vi "BuildTriggerArray for Closed IPG.vi"(0 "CBC Trigger Level":dbl, 1 "Load Resistance (Ohms)":dbl, 2 "Target Stim Current (Amps)":dbl, 3 "Krec Value":i32, 4 "Recovery Mode (T=Active)":bool) -> (5 "Pulse Triggers":T1(array[cluster]))   [LabVIEW 2010]
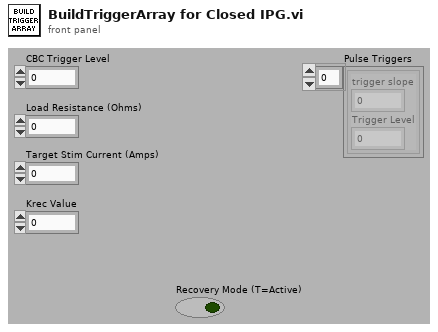
[diagram p1: front panel]
types:
  T1 = cluster{"trigger slope":u16, "Trigger Level":dbl}[]
  T2 = cluster{"trigger slope":u16, "Trigger Level":dbl}
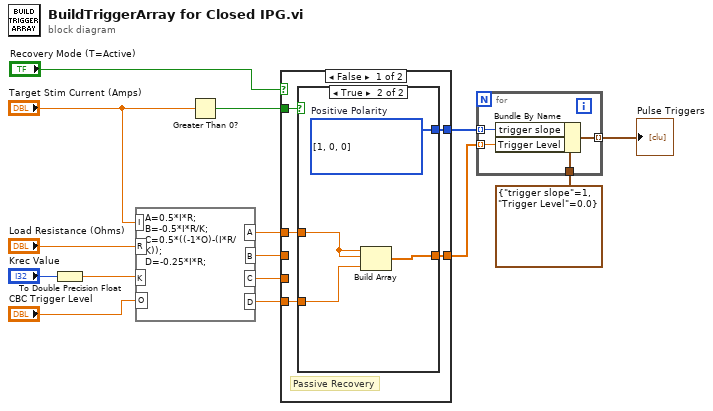
[diagram p0: block diagram]
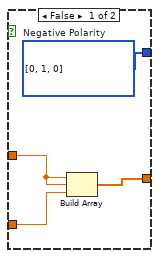
[diagram p2: hidden frame]
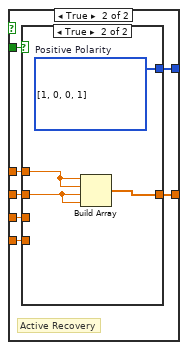
[diagram p3: hidden frame]
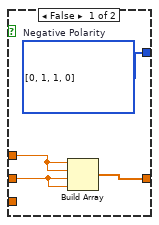
[diagram p4: hidden frame]
diagram:
  n1 = To Double Precision Float(number="Krec Value") -> (double precision float=w8:dbl)
  n2 = formula code="A=0.5*I*R;\nB=-0.5*I*R/K;\nC=0.5*((-1*O)-(I*R/K));\nD=-0.25*I*R;"("R"="Load Resistance (Ohms)", "I"="Target Stim Current (Amps)", "K"=w8, "O"="CBC Trigger Level") -> ("A"=w5:dbl, "B"=w4:dbl, "C"=w3:dbl, "D"=w2:dbl)
  n3 = Greater Than 0?(x="Target Stim Current (Amps)") -> (x > 0?=w14:bool)
  n4 = case shown="False" "Recovery Mode (T=Active)" {
    tunnel: [w19 w35] -> w11
    tunnel: w14 -> [w20 w34]
    tunnel: w5 -> [w18 w33]
    tunnel: w4 -> [_ w32]
    tunnel: w3 -> [_ w31]
    tunnel: w2 -> [w17 w30]
    tunnel: [w16 w29] -> w1
    frame False {
      # "Passive Recovery"
      n5 = case shown="True" w20 {
        tunnel: [w24 w28] -> w19
        tunnel: w18 -> [w23 w27]
        tunnel: w17 -> [w22 w26]
        tunnel: [w21 w25] -> w16
        frame False {
          w24 = u16[] [0, 1, 0] items=["Falling Edge", "Rising Edge"]  # Negative Polarity
          n6 = Build Array(w23, w23, w22) -> (w21:dbl[])
        }
        frame True {
          w28 = u16[] [1, 0, 0] items=["Falling Edge", "Rising Edge"]  # Positive Polarity
          n7 = Build Array(w27, w27, w26) -> (w25:dbl[])
        }
      }
    }
    frame True {
      # "Active Recovery"
      n8 = case shown="True" w34 {
        tunnel: [w39 w43] -> w35
        tunnel: w33 -> [w38 w42]
        tunnel: w32 -> [w36 w40]
        tunnel: w31 -> [_ _]
        tunnel: w30 -> [_ _]
        tunnel: [w37 w41] -> w29
        frame False {
          w39 = u16[] [0, 1, 1, 0] items=["Falling Edge", "Rising Edge"]  # Negative Polarity
          n9 = Build Array(w38, w38, w36, w36) -> (w37:dbl[])
        }
        frame True {
          w43 = u16[] [1, 0, 0, 1] items=["Falling Edge", "Rising Edge"]  # Positive Polarity
          n10 = Build Array(w42, w42, w40, w40) -> (w41:dbl[])
        }
      }
    }
  }
  n11 = for {
    tunnel: T2 {"trigger slope"=1, "Trigger Level"=0.0} -> [w47]
    tunnel: w11 -> [w46] mode=indexing
    tunnel: w1 -> [w45] mode=indexing
    tunnel: [w44] -> w13 mode=indexing
    n12 = Bundle By Name(cluster=w47, "trigger slope"=w46, "Trigger Level"=w45) -> (w44:T2)
  }
  "Pulse Triggers" <- w13
